vi "Create Request Helper.vi"(8 "Create Request Argument":T2, 11 "Module Data":T1) -> (0 "Create Request (Reply Payload)":T3, 1 "Message":string, 3 "Module Data out":T1)   [LabVIEW 2024, in "DQMH Power Requests.lvlib"]
doc: "<b>Note:</b> This VI was modified by the <b>Validate DQMH Module</b> tool to turn off automatic error handling.\n\n<b>Note:</b> This VI was modified by the <b>Validate DQMH Module</b> tool to be shared clone reentrant."
uses:
  DQMH Power Requests.lvlib
  Create Request (Reply Payload)--cluster.ctl
  Create Request Argument--cluster.ctl
  Module Data--cluster.ctl
  Power-Requests/Power Availabilty Requests/Type Defs/Power Availiability Requests Functions.ctl
  Power-Requests/Power Availabilty Requests/Type Defs/Power Request Type.ctl
  <vilib>/ErrorRing/Error Ring.xnode
  Power-Requests/Power Requests.lvlib
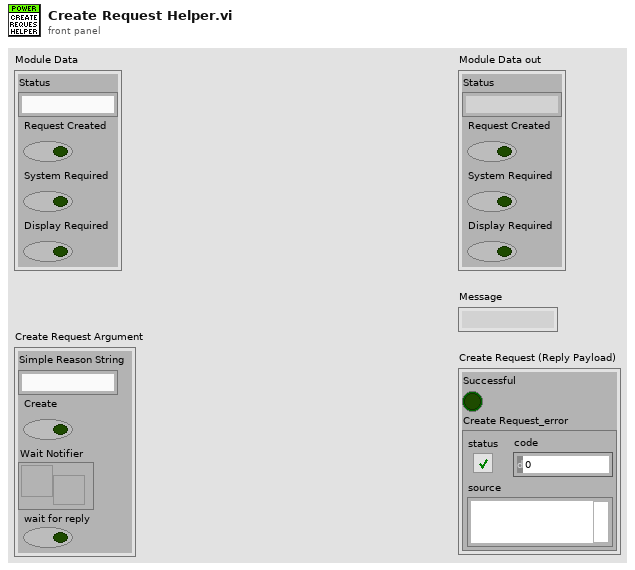
[diagram p1: front panel]
types:
  T1 = typedef "DQMH Power Requests.lvlib/Module Data--cluster.ctl" = cluster{"Status":string, "Request Created":bool, "System Required":bool, "Display Required":bool}
  T2 = typedef "DQMH Power Requests.lvlib/Create Request Argument--cluster.ctl" = cluster{"Simple Reason String":string, "Create":bool, "Wait Notifier":refnum<notifier>, "wait for reply":bool}
  T3 = typedef "DQMH Power Requests.lvlib/Create Request (Reply Payload)--cluster.ctl" = cluster{"Successful":bool, "Create Request_error":errorcluster}
  T4 = typedef "Power Requests.lvlib/Power Availiability Requests Functions.ctl" = enum32{"Power Create Request", "Power Set Request", "Power Clear Request", "Close Handle"}
  T5 = typedef "Power Requests.lvlib/Power Request Type.ctl" = enum32{"Power Request Display Required", "Power Request System Required", "Power Request Away Mode Required", "Power Request Execution Required"}
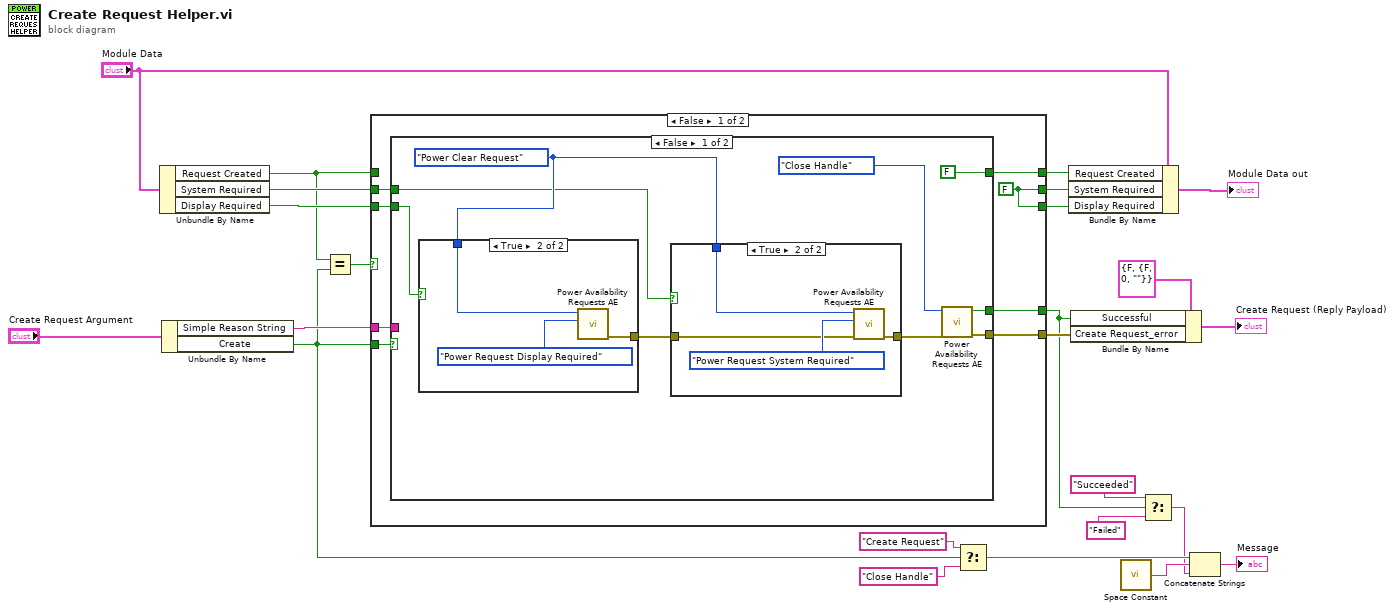
[diagram p0: block diagram]
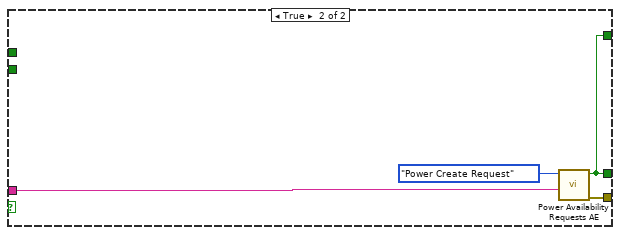
[diagram p4: hidden frame]
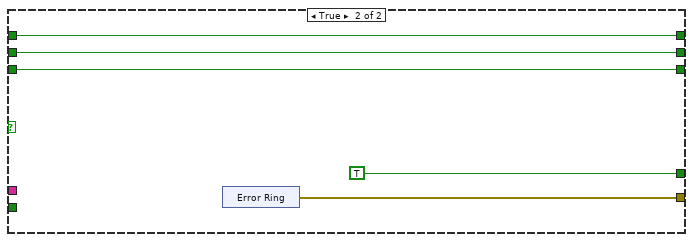
[diagram p5: hidden frame]
diagram:
  n1 = Unbundle By Name("Module Data") -> ("Request Created"=w12:bool, "System Required"=w16:bool, "Display Required"=w15:bool)
  n2 = Unbundle By Name("Create Request Argument") -> ("Simple Reason String"=w13:string, "Create"=w2:bool)
  n3 = Equal?(x=w12, y=w2) -> (x = y?=w11:bool)
  n4 = case shown="False" w11 {
    tunnel: [w32 w57] -> w14
    tunnel: [w31 TRUE] -> w1
    tunnel: w13 -> [w30 _]
    tunnel: w2 -> [w29 _]
    tunnel: w12 -> [_ w56]
    tunnel: [w28 w56] -> w19
    tunnel: w15 -> [w26 w55]
    tunnel: [w27 w55] -> w17
    tunnel: w16 -> [w25 w54]
    tunnel: [w27 w54] -> w18
    frame False {
      w27 = FALSE
      n5 = case shown="False" w29 {
        tunnel: [w40 w53] -> w32
        tunnel: [w41 w50] -> w31
        tunnel: w30 -> [_ w51]
        tunnel: [FALSE w50] -> w28
        tunnel: w26 -> [w37 _]
        tunnel: w25 -> [w35 _]
        frame False {
          w36 = Power_Availiability_Requests_Functions."Power Clear Request" ("Power Availability Requests Functions")
          n6 = case shown="True" w37 {
            tunnel: w36 -> [_ w49]
            tunnel: [_ w47] -> w33
            frame False {
            }
            frame True {
              n7 = call "Power Availability Requests AE.vi"("Power Request Type"=Power_Request_Type."Power Request Display Required", "Power Availability Requests Functions"=w49) -> ("error out"=w47:errorcluster)  [unwired: 8 in, 1 out]
            }
          }
          n8 = case shown="True" w35 {
            tunnel: w36 -> [_ w46]
            tunnel: [w42 w45] -> w34
            tunnel: w33 -> [w42 w43]
            frame False {
            }
            frame True {
              n9 = call "Power Availability Requests AE.vi"("error in (no error)"=w43, "Power Request Type"=Power_Request_Type."Power Request System Required", "Power Availability Requests Functions"=w46) -> ("error out"=w45:errorcluster)  [unwired: 7 in, 1 out]
            }
          }
          n10 = call "Power Availability Requests AE.vi"("error in (no error)"=w34, "Power Availability Requests Functions"=Power_Availiability_Requests_Functions."Close Handle") -> ("error out"=w40:errorcluster, "Success?"=w41:bool)  [unwired: 8 in]
        }
        frame True {
          n11 = call "Power Availability Requests AE.vi"("Simple Reason String"=w51, "Power Availability Requests Functions"=Power_Availiability_Requests_Functions."Power Create Request") -> ("error out"=w53:errorcluster, "Success?"=w50:bool)  [unwired: 8 in]
        }
      }
    }
    frame True {
      n12 = xnode "Error Ring"() -> ("error out"=w57:errorcluster)
    }
  }
  n13 = Select(t="Create Request", s=w2, f="Close Handle") -> (s? t:f=w7:string)
  n14 = Bundle By Name(cluster="Module Data", "Request Created"=w19, "System Required"=w18, "Display Required"=w17) -> (→"Module Data out":T1)
  n15 = Bundle By Name(cluster=T3 {"Successful"=FALSE, "Create Request_error"={"status"=FALSE, "code"=0, "source"=""}} ("Create Request (Reply Payload)"), "Successful"=w1, "Create Request_error"=w14) -> (→"Create Request (Reply Payload)":T3)
  n16 = call <vilib>:"Space Constant.vi"() -> ("String"=w10:string)
  n17 = Select(t="Succeeded", s=w1, f="Failed") -> (s? t:f=w6:string)
  n18 = Concatenate Strings(w7, w10, w6) -> (→"Message":string)
